vi "CmdSetOman_ParseArg.vi"(10 "number of params":i32, 11 "args in":string) -> (1 "value":string, 2 "key":string, 3 "remaining args":string)   [LabVIEW 2016]
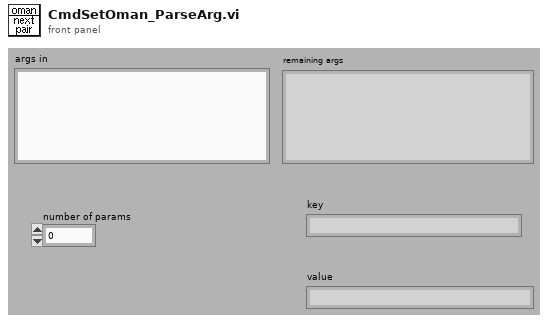
[diagram p1: front panel]
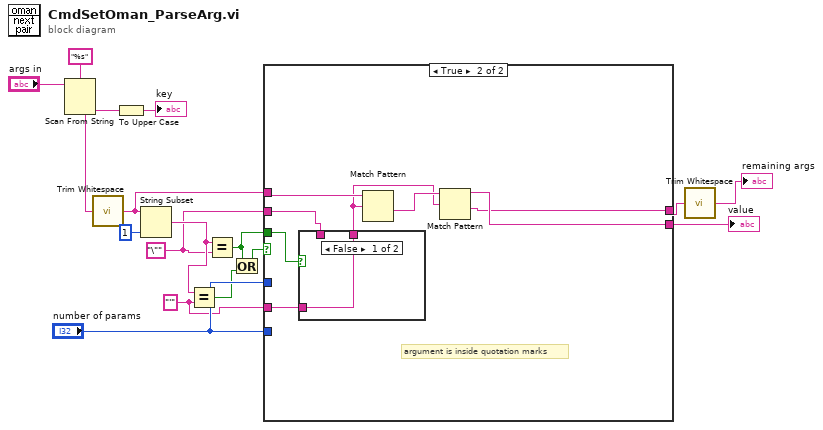
[diagram p0: block diagram]
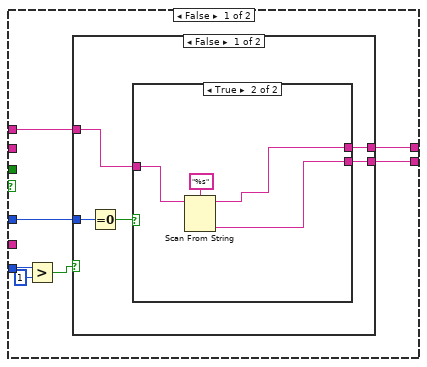
[diagram p2: hidden frame]
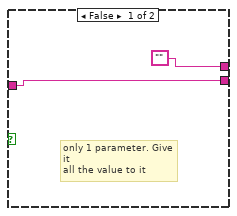
[diagram p3: hidden frame]
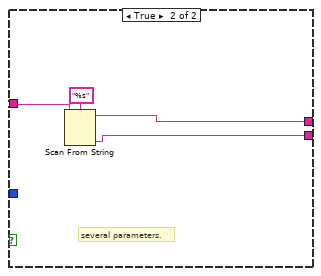
[diagram p4: hidden frame]
diagram:
  w1 = "'" ("y")
  w2 = "\"" ("y")
  n1 = Scan From String(format string="%s", input string="args in") -> (remaining string=w14:string, output 1=w15:string)  [unwired: 2 in, 3 out]
  n2 = call <vilib>:"Trim Whitespace.vi"("string"=w14) -> ("trimmed string"=w12:string)  [unwired: 1 in]
  n3 = To Upper Case(1:w15) -> (0:→"key":string)
  n4 = String Subset(string=w12, length (rest)=1 ("length (rest)")) -> (substring=w5:string)  [unwired: 1 out]
  n5 = Equal?(x=w5, y=w1) -> (x = y?=w6:bool)
  n6 = Equal?(x=w5, y=w2) -> (x = y?=w3:bool)
  n7 = Or(x=w3, y=w6) -> (x .or. y?=w4:bool)
  n8 = case shown="True" w4 {
    tunnel: w12 -> [w24 w47]
    tunnel: [w23 w45] -> w11
    tunnel: [w22 w44] -> w10
    tunnel: "number of params" -> [w21 _]
    tunnel: "number of params" -> [w18 _]
    tunnel: w3 -> [_ w43]
    tunnel: w2 -> [_ w42]
    tunnel: w1 -> [_ w40]
    frame False {
      n9 = Greater?(x=w21, y=1) -> (0:w19:bool)
      n10 = case shown="False" w19 {
        tunnel: w24 -> [w26 w39]
        tunnel: [w25 w37] -> w23
        tunnel: [w29 w36] -> w22
        tunnel: w18 -> [w28 _]
        frame False {
          n11 = Equal To 0?(x=w28) -> (x = 0?=w27:bool)
          n12 = case shown="True" w27 {
            tunnel: ["" w32] -> w29
            tunnel: w26 -> [w31 w34]
            tunnel: [w31 w33] -> w25
            frame False {
              # "only 1 parameter. Give it\nall the value to it"
            }
            frame True {
              n13 = Scan From String(format string="%s", input string=w34) -> (remaining string=w32:string, output 1=w33:string)  [unwired: 2 in, 3 out]
            }
          }
        }
        frame True {
          # "several parameters."
          n14 = Scan From String(format string="%s", input string=w39) -> (remaining string=w36:string, output 1=w37:string)  [unwired: 2 in, 3 out]
        }
      }
    }
    frame True {
      # "argument is inside quotation marks"
      n15 = case shown="False" w43 {
        tunnel: w42 -> [_ w49]
        tunnel: [w48 w49] -> w41
        tunnel: w40 -> [w48 _]
        frame False {
        }
        frame True {
        }
      }
      n16 = Match Pattern(string=w47, regular expression=w41) -> (after substring=w46:string)  [unwired: 4 out]
      n17 = Match Pattern(string=w46, regular expression=w41) -> (before substring=w45:string, after substring=w44:string)  [unwired: 3 out]
    }
  }
  "value" <- w11
  n18 = call <vilib>:"Trim Whitespace.vi"("string"=w10) -> ("trimmed string"=→"remaining args":string)  [unwired: 1 in]
